vi "TrackStack.vi"(8 "WindDirection":dbl, 9 "StackPosition (at 0deg)":sgl[](array[numeric]), 11 "Demanded Position":sgl[](array[numeric])) -> (1 "CurrentStackPosition":sgl[](array[numeric]) format="%.2f", 3 "Adjusted Position":sgl[](array[numeric]) format="%.2f")   [LabVIEW 2015]
panel:
  in  "Menu Ring":enum16{"Track X and Y", "Track Y only"}(ring)
  # "This VI takes a position demand relative to 0,0, and transposes it to an alternative origin, which rotates with the turntable- e.g. an off-centre stack..."
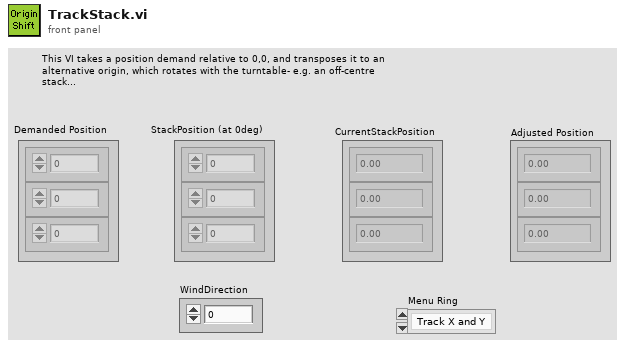
[diagram p1: front panel]
types:
  T1 = cluster{"StackPosition (at 0deg)[0]":sgl, "StackPosition (at 0deg)[1]":sgl, "StackPosition (at 0deg)[2]":sgl}
  T2 = cluster{dbl, dbl, "StackPosition (at 0deg)[2]":sgl}
  T3 = cluster{sgl, sgl, "StackPosition (at 0deg)[2]":sgl}
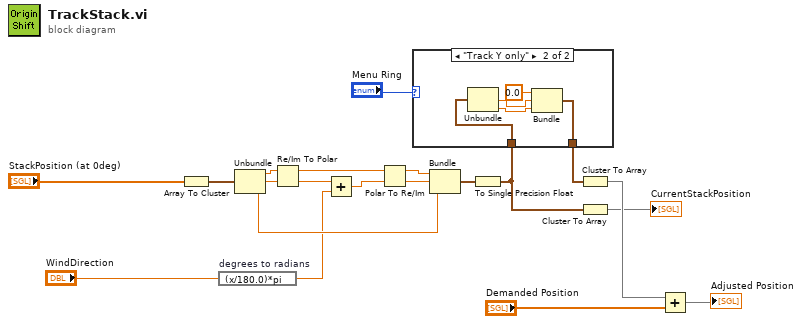
[diagram p0: block diagram]
diagram:
  n1 = Array To Cluster(array="StackPosition (at 0deg)") -> (cluster=w17:T1)
  n2 = expression code="(x/180.0)*pi" "degrees to radians"("WindDirection") -> (w8:dbl)
  n3 = Unbundle(w17) -> ("StackPosition (at 0deg)[0]"=w12:sgl, "StackPosition (at 0deg)[1]"=w13:sgl, "StackPosition (at 0deg)[2]"=w14:sgl)
  n4 = Re/Im To Polar(2:w13, 3:w12) -> (0:w19:sgl, 1:w20:sgl)
  n5 = Add(x=w19, y=w8) -> (x+y=w11:dbl)
  n6 = Polar To Re/Im(2:w11, 3:w20) -> (0:w15:dbl, 1:w16:dbl)
  n7 = Bundle(w16, w15, "StackPosition (at 0deg)[2]"=w14) -> (w10:T2)  [unwired: 1 in]
  n8 = To Single Precision Float(number=w10) -> (single precision float=w2:T3)
  n9 = case shown="\"Track Y only\"" "Menu Ring" {
    tunnel: [w21 w26] -> w3
    tunnel: w2 -> [w21 w24]
    frame "Track X and Y", Default {
    }
    frame "Track Y only" {
      n10 = Unbundle(w24) -> (w23:sgl, "StackPosition (at 0deg)[2]"=w22:sgl)  [unwired: 1 out]
      n11 = Bundle(sgl 0.0, w23, "StackPosition (at 0deg)[2]"=w22) -> (w26:T3)  [unwired: 1 in]
    }
  }
  n12 = Cluster To Array(cluster=w3) -> (array=w7:sgl[])
  n13 = Cluster To Array(cluster=w2) -> (array=→"CurrentStackPosition":sgl[])
  n14 = Add(x=w7, y="Demanded Position") -> (x+y=→"Adjusted Position":sgl[])
